vi "Historian.vi"() -> ()   [LabVIEW 2018]
uses:
  <vilib>/measure/NI_MABase.lvlib
panel:
  out "Number Data Points Collected":dbl
  out "Next Data Grab Time":dbl
  out "Sample Rate":dbl
  out "Current Data Point":dbl
  out "Current Relative Time":dbl
  out "Run Indicator":bool
  in  "stop":bool
  in  "Runtime Step Rate (s)":dbl
  out "Incoming Data (Static Right Now)":waveform(dbl)(graph)
  in  "Save The DATA!":bool
  in  "Over Number of Seconds":dbl
  in  "Number of Samples":dbl
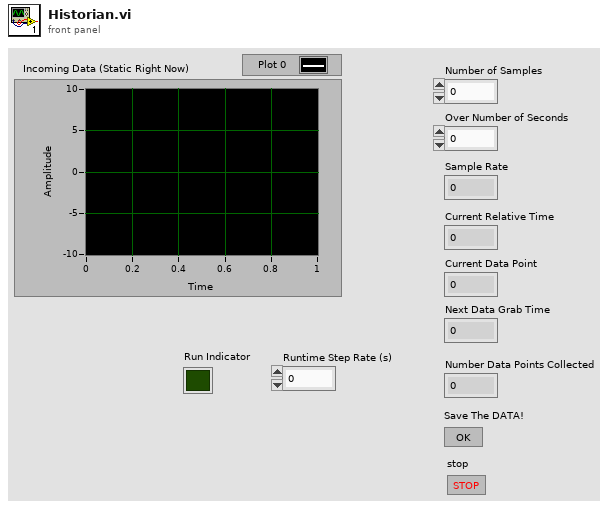
[diagram p1: front panel]
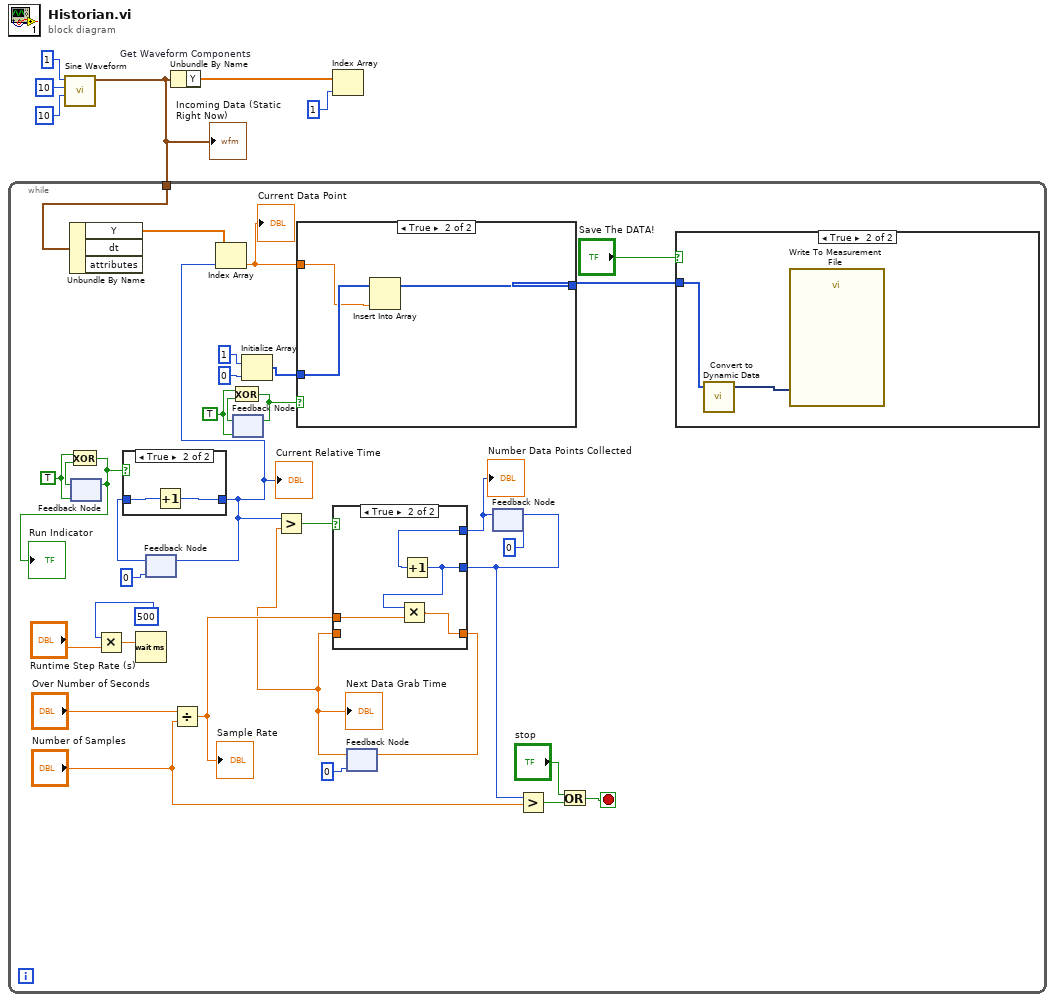
[diagram p0: block diagram]
diagram:
  n1 = call <vilib>:"Sine Waveform.vi"("phase"=10, "amplitude"=10, "frequency"=1) -> ("signal out"=w1:waveform(dbl))  [unwired: 7 in, 1 out]
  "Incoming Data (Static Right Now)" <- w1
  n2 = while {
    tunnel: w1 -> [w35]
    stop <- w7 stop-if-true
    w26 = TRUE
    w33 = TRUE
    n3 = Unbundle By Name(w35) -> ("Y"=w34:dbl[])  [unwired: 2 out]
    n4 = feedback #1(w33) -> (w32:bool)
    n5 = Exclusive Or(1:w32, 2:w33) -> (0:w29:bool)
    "Run Indicator" <- w29
    n6 = feedback-in #1(w29) -> ()
    n7 = Multiply(x=500, y="Runtime Step Rate (s)") -> (x*y=w38:dbl)
    n8 = Wait (ms)(milliseconds to wait=w38) -> ()  [unwired: 1 out]
    n9 = feedback #2(0) -> (w31:i32)
    n10 = case shown="True" w29 {
      tunnel: w31 -> [w50 w52]
      tunnel: [w50 w51] -> w17
      frame False {
      }
      frame True {
        n11 = Increment(x=w52) -> (x+1=w51:i32)
      }
    }
    "Current Relative Time" <- w17
    n12 = feedback-in #2(w17) -> ()
    n13 = Divide(x="Over Number of Seconds", y="Number of Samples") -> (x/y=w15:dbl)
    "Sample Rate" <- w15
    n14 = Index Array(array=w34, index=w17) -> (element=w21:dbl)
    "Current Data Point" <- w21
    n15 = feedback #3(w26) -> (w25:bool)
    n16 = Exclusive Or(1:w25, 2:w26) -> (0:w24:bool)
    n17 = feedback-in #3(w24) -> ()
    n18 = Initialize Array(1, 0) -> (w23:i32[])
    n19 = case shown="True" w24 {
      tunnel: w21 -> [_ w48]
      tunnel: w23 -> [w46 w49]
      tunnel: [w46 w47] -> w22
      frame False {
      }
      frame True {
        n20 = Insert Into Array(array=w49, new element=w48) -> (w47:i32[])  [unwired: 1 in]
      }
    }
    n21 = feedback #4(0) -> (w14:dbl)
    "Next Data Grab Time" <- w14
    n22 = Greater?(x=w17, y=w14) -> (0:w16:bool)
    n23 = feedback #5(0) -> (w12:i32)
    "Number Data Points Collected" <- w12
    n24 = case shown="True" w16 {
      tunnel: w14 -> [w41 _]
      tunnel: [w41 w44] -> w18
      tunnel: w15 -> [_ w45]
      tunnel: w12 -> [w40 w43]
      tunnel: [w40 w42] -> w11
      frame False {
      }
      frame True {
        n25 = Increment(x=w43) -> (x+1=w42:i32)
        n26 = Multiply(x=w42, y=w45) -> (x*y=w44:dbl)
      }
    }
    n27 = feedback-in #4(w18) -> ()
    n28 = feedback-in #5(w11) -> ()
    n29 = Greater?(x=w11, y="Number of Samples") -> (0:w9:bool)
    n30 = Or(x="stop", y=w9) -> (x .or. y?=w7:bool)
    n31 = case shown="True" "Save The DATA!" {
      tunnel: w22 -> [_ w54]
      frame False {
      }
      frame True {
        n32 = call "Convert to Dynamic Data"("Array"=w54) -> ("Dynamic Data Type"=w53:dynamicdata)  [unwired: 3 in]
        n33 = call "Write To Measurement File"("Signals"=w53) -> ()  [unwired: 16 in, 3 out]
      }
    }
  }
  n34 = Unbundle By Name "Get Waveform Components"(w1) -> ("Y"=w6:dbl[])
  n35 = Index Array "Index Array"(array=w6, index=1) -> ()  [unwired: 1 out]
